vi "zadanie_2.vi"() -> ()   [LabVIEW 2020]
panel:
  in  "stop":bool
  out "suma":dbl
  in  "zadane n":dbl
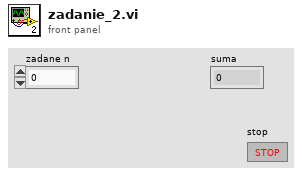
[diagram p1: front panel]
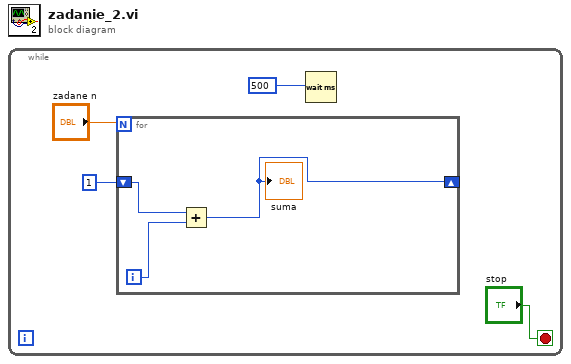
[diagram p0: block diagram]
diagram:
  n1 = while {
    stop <- "stop" stop-if-true
    n2 = for {
      N: "zadane n" -> [_]
      shift-right: [w5] -> _
      shift-left: 1 -> [w7]
      i -> [w6]
      n3 = Add(x=w7, y=w6) -> (x+y=w5:i32)
      "suma" <- w5
    }
    n4 = Wait (ms)(milliseconds to wait=500) -> ()  [unwired: 1 out]
  }
